vi "Test-CreateClose.vi"() -> ()   [LabVIEW 2009]
uses:
  Clients/H5F-File/H5F_ACC.ctl
panel:
  out "file_id":i32
  out "status":i32
  in  "flags":T1[](array[typedef])
  in  "filename":path
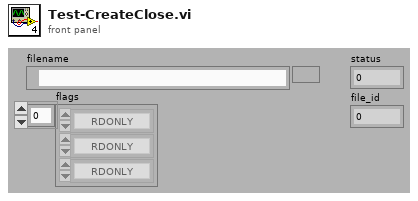
[diagram p1: front panel]
types:
  T1 = typedef "H5F_ACC.ctl" = enum16{"RDONLY", "RDWR", "TRUNC", "EXCL", "DEBUG", "CREAT"}
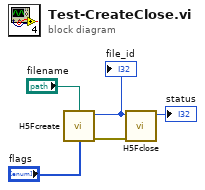
[diagram p0: block diagram]
diagram:
  n1 = call "H5Fcreate.vi"("filename"="filename", "flags"="flags") -> ("file_id"=w5:i32, "error out"=w4:errorcluster)  [unwired: 6 in]
  "file_id" <- w5
  n2 = call "H5Fclose.vi"("error in (no error)"=w4, "file_id"=w5) -> ("status"=→"status":i32)  [unwired: 8 in, 1 out]
